vi "Error Massege.vi"(0 "Boolean":bool, 1 "Error M Auto":string) -> (7 "Cluster":cluster{"Boolean":bool, "Error":string})   [LabVIEW 2015]
panel:
  in  "stop":bool
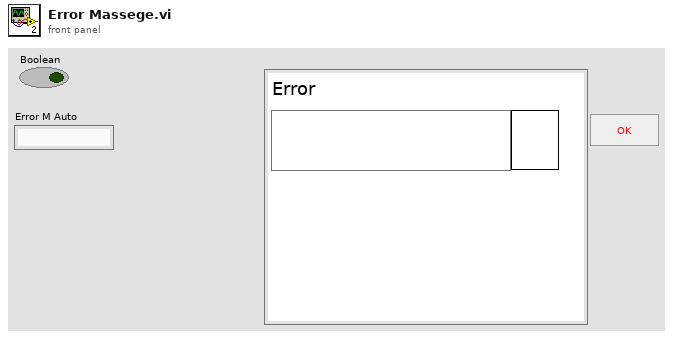
[diagram p1: front panel]
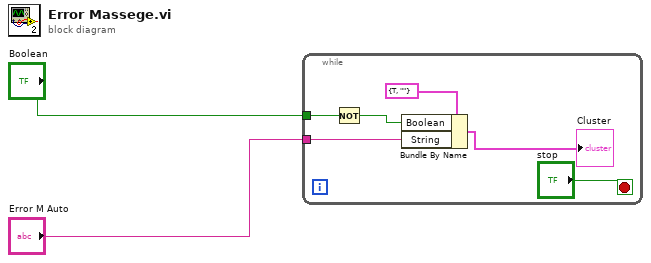
[diagram p0: block diagram]
diagram:
  n1 = while {
    tunnel: "Boolean" -> [w7]
    tunnel: "Error M Auto" -> [w5]
    stop <- "stop" stop-if-true
    n2 = Not(x=w7) -> (.not. x?=w6:bool)
    n3 = Bundle By Name(cluster=cluster{"Boolean":bool, "String":string} {"Boolean"=TRUE, "String"=""} ("Cluster 2"), "Boolean"=w6, "String"=w5) -> (→"Cluster":cluster{"Boolean":bool, "String":string})
  }
